vi "KM101_SerialCreat.vi"(9 "HWSerialNum":i32=97100662, 10 "reference in":refnum<k7>) -> (2 "reference out":refnum<k7>)   [LabVIEW 2018, in "KIM101lib.lvlib"]
uses:
  KIM101lib.lvlib
  <vilib>/Utility/error.llb/DialogType.ctl
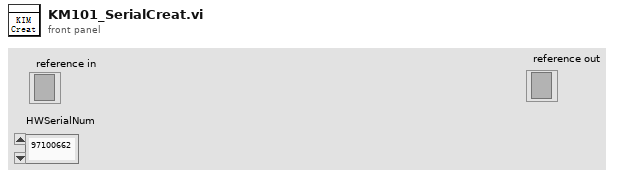
[diagram p1: front panel]
types:
  T1 = typedef "DialogType.ctl" = u16
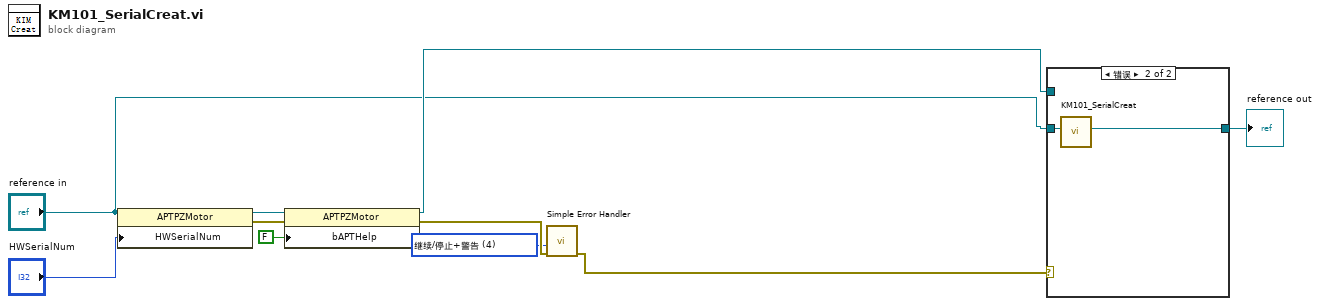
[diagram p0: block diagram]
diagram:
  w1 = T1 4 items=["无对话框", "确定信息", "继续或停止信息", "确定信息＋警告", "继续/停止+警告"] ("type of dialog (OK msg:1)")
  n1 = property class="APTPZMotor"(reference="reference in", "HWSerialNum"="HWSerialNum") -> (reference out=w8:refnum<k7>, error out=w7:errorcluster)  [unwired: 1 in]
  n2 = property class="APTPZMotor"(reference=w8, error in=w7, "bAPTHelp"=FALSE) -> (reference out=w5:refnum<k7>, error out=w3:errorcluster)
  n3 = call <vilib>:"Simple Error Handler.vi"("type of dialog (OK msg:1)"=w1, "error in (no error)"=w3) -> ("error out"=w2:errorcluster)  [unwired: 3 in, 4 out]
  n4 = case shown="错误" w2 {
    tunnel: w5 -> [w11 _]
    tunnel: [w11 w12] -> w6
    tunnel: "reference in" -> [_ w13]
    frame No Error {
    }
    frame Error {
      n5 = call "KM101_SerialCreat.vi"("reference in"=w13) -> ("reference out"=w12:refnum<k7>)  [unwired: 10 in]
    }
  }
  "reference out" <- w6
